vi "MAG STAB.vi"(0 "VISA In":refnum<visa-resource-name>, 1 "MagQ":refnum<queue>, 2 "ScanQ":refnum<queue>, 3 "PSU Status In":T1 {"Trip Current" format="%.3f"; "Trip Field" format="%.4f"; "Voltage" format="%.2f"; "Field Constant" format="%.6f"; "MID Setpoint (T)" format="%.4f"; "MID Setpoint (A)" format="%.3f"; "MAX Setpoint (T)" format="%.4f"; "MAX Setpoint (A)" format="%.3f"; "Heater Voltage" format="%.2f"; "V Limit (V)" format="%.2f"; "Ramp Rate (A/s)" format="%.3f"; "Output (A)" format="%.3f"; "Output (T)" format="%.4f"; "Persistent Current" format="%.3f"; "Persistent Field" format="%.4f"}, 4 "P-Mode Ramp Rate (A/s)":dbl, 5 "Error out":errorcluster, 6 "Boolean":bool) -> (14 "VISA Out":refnum<visa-resource-name>, 15 "MagQ":refnum<queue>, 16 "PSU Status Out":T1 {"Trip Current" format="%.3f"; "Trip Field" format="%.4f"; "Voltage" format="%.2f"; "Field Constant" format="%.6f"; "MID Setpoint (T)" format="%.4f"; "MID Setpoint (A)" format="%.3f"; "MAX Setpoint (T)" format="%.4f"; "MAX Setpoint (A)" format="%.3f"; "Heater Voltage" format="%.2f"; "V Limit (V)" format="%.2f"; "Ramp Rate (A/s)" format="%.3f"; "Output (A)" format="%.3f"; "Output (T)" format="%.4f"; "Persistent Current" format="%.3f"; "Persistent Field" format="%.4f"}, 19 "error out":errorcluster)   [LabVIEW 2025]
uses:
  Labview-File/STM-Auto-Project Testing/STM-Auto-Project (Trial 2)/QMH CTLS/Scan_Params (QMH).ctl
  <instrlib>/SMS LabVIEW Drivers/Source Code/Cryogenic Ltd SMSXXX.lvlib
  <instrlib>/SMS LabVIEW Drivers/Source Code/Public/PSU Status.ctl
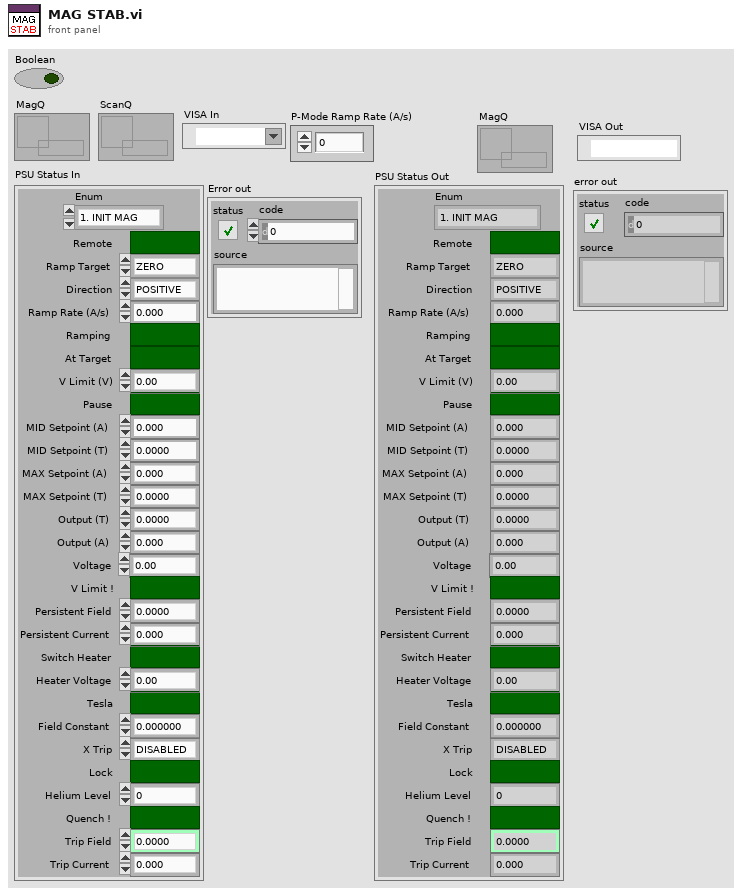
[diagram p1: front panel]
types:
  T1 = typedef "Cryogenic Ltd SMSXXX.lvlib/PSU Status.ctl" = cluster{"Ramp Target":enum16{"ZERO", "MID", "MAX"}, "Pause":bool, "Switch Heater":bool, "Persistent Field":dbl, "Persistent Current":dbl, "Tesla":bool, "Output (T)":dbl, "Output (A)":dbl, "X Trip":enum16{"DISABLED", "ENABLED", "ACTIVE"}, "Ramp Rate (A/s)":dbl, "V Limit (V)":dbl, "Heater Voltage":dbl, "MAX Setpoint (A)":dbl, "MAX Setpoint (T)":dbl, "MID Setpoint (A)":dbl, "MID Setpoint (T)":dbl, "Lock":bool, "Field Constant":dbl, "Remote":bool, "Direction":enum16{"POSITIVE", "NEGATIVE", "OPEN", "UNIPOLAR"}, "Helium Level":u16, "Quench !":bool, "Voltage":dbl, "V Limit !":bool, "Ramping":bool, "At Target":bool, "Trip Field":dbl, "Trip Current":dbl, "Enum":enum16{"1. INIT MAG", "2. MAG ON ", "3. MAG_STAB", "4. MAG IDLE", "5. NEXT FIELD", "6. MAG OFF (Reset)"}}
  T2 = enum16{"1. INIT MAG", "2. MAG ON", "3. MAG_STAB", "4. MAG IDLE", "5. PREP NEXT FIELD", "6. APPLY NEXT FIELD", "7. PREP OFF", "8. MAG OFF (Reset)"}
  T3 = enum16{"1. BIAS", "2. INIT_SCAN", "3. SCAN_IDLE", "4. INTER_SCAN", "5. NEW_COORDS_&_FRAME", "6. FINAL_SCAN", "7. POLL BIAS ", "8. Z-CONT.", "9. STOP"}
  T4 = typedef "Scan_Params (QMH).ctl" = cluster{"Setpoint (I)":dbl[], "Bias (V)":dbl[], "Number of scans":u8, "Port number (3364)":u32, "Avoid zero threshold (V)":dbl, "Current State":enum16{"1. BIAS", "2. INIT_SCAN", "3. SCAN_IDLE", "4. INTER_SCAN", "5. NEW_COORDS_&_FRAME", "6. FINAL_SCAN", "7. STOP"}}
  T5 = enum16{"RAMP TO ZERO", "RAMP TO MID", "RAMP TO MAX"}
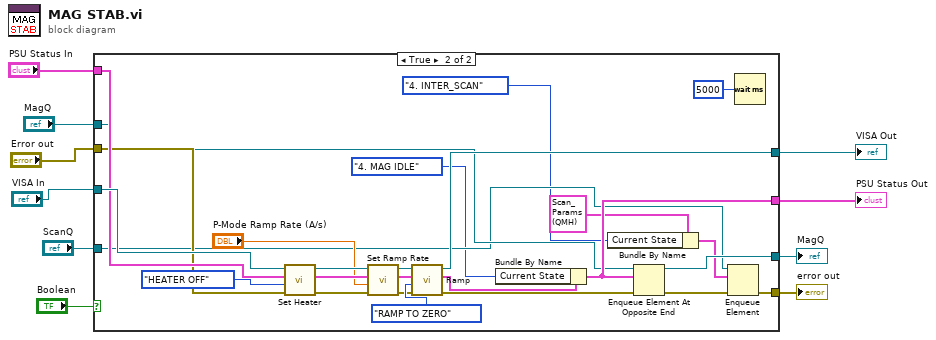
[diagram p0: block diagram]
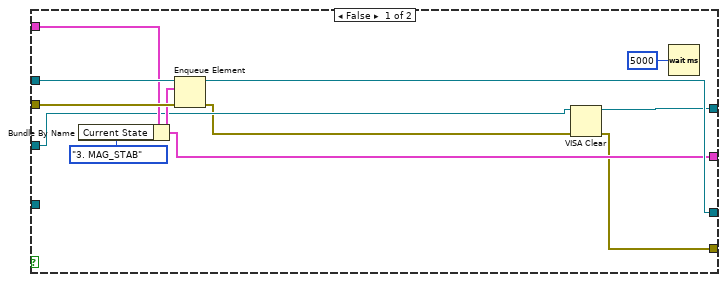
[diagram p2: hidden frame]
diagram:
  n1 = case shown="True" "Boolean" {
    tunnel: [w11 w27] -> w2
    tunnel: [w21 w46] -> w3
    tunnel: [w16 w40] -> w4
    tunnel: [w14 w43] -> w5
    tunnel: "VISA In" -> [w15 w39]
    tunnel: "PSU Status In" -> [w17 w38]
    tunnel: "Error out" -> [w18 w37]
    tunnel: "MagQ" -> [w19 w36]
    tunnel: "ScanQ" -> [_ w26]
    frame False {
      n2 = Bundle By Name(cluster=w17, "Current State"=T2."3. MAG_STAB") -> (w16:T1)
      n3 = Enqueue Element(queue=w19, element=w16, error in (no error)=w18) -> (queue out=w21:refnum<queue>, error out=w12:errorcluster)  [unwired: 1 in, 1 out]
      n4 = VISA Clear(VISA resource name=w15, error in (no error)=w12) -> (VISA resource name out=w14:refnum<visa-resource-name>, error out=w11:errorcluster)
      n5 = Wait (ms)(milliseconds to wait=u32 5000) -> ()  [unwired: 1 out]
    }
    frame True {
      n6 = call <instrlib>:"Set Heater.vi"("Error in (no error)"=w37, "Heater (On/Off)"=enum16{"HEATER OFF", "HEATER ON"}."HEATER OFF", "PSU Status In"=w38, "VISA Resource Name In"=w39) -> ("Error out"=w35:errorcluster, "PSU Status Out"=w33:T1, "VISA Resource Name Out"=w34:refnum<visa-resource-name>)  [unwired: 4 in, 1 out]
      n7 = call <instrlib>:"Set Ramp Rate.vi"("Error in (no error)"=w35, "Ramp Rate (A/s)"="P-Mode Ramp Rate (A/s)", "PSU Status In"=w33, "VISA Resource Name In"=w34) -> ("Error out"=w30:errorcluster, "PSU Status Out"=w32:T1, "VISA Resource Name Out"=w31:refnum<visa-resource-name>)  [unwired: 4 in, 1 out]
      n8 = call <instrlib>:"Ramp.vi"("Error in (no error)"=w30, "Ramp Target"=T5."RAMP TO ZERO", "PSU Status In"=w32, "VISA Resource Name In"=w31) -> ("Error out"=w42:errorcluster, "PSU Status Out"=w41:T1, "VISA Resource Name Out"=w43:refnum<visa-resource-name>)  [unwired: 4 in, 1 out]
      n9 = Bundle By Name(cluster=w41, "Current State"=T2."4. MAG IDLE") -> (w40:T1)
      n10 = Bundle By Name(cluster=T4 {"Setpoint (I)"=[], "Bias (V)"=[], "Number of scans"=1, "Port number (3364)"=3364, "Avoid zero threshold (V)"=0.004999999888241291, "Current State"=enum."1. BIAS"} ("element"), "Current State"=T3."4. INTER_SCAN") -> (w24:T4)
      n11 = Enqueue Element At Opposite End(queue=w36, element=w40, error in (no error)=w42) -> (queue out=w46:refnum<queue>, error out=w28:errorcluster)  [unwired: 1 in, 1 out]
      n12 = Enqueue Element(queue=w26, element=w24, error in (no error)=w28) -> (error out=w27:errorcluster)  [unwired: 1 in, 2 out]
      n13 = Wait (ms)(milliseconds to wait=u32 5000) -> ()  [unwired: 1 out]
    }
  }
  "VISA Out" <- w5
  "PSU Status Out" <- w4
  "MagQ" <- w3
  "error out" <- w2
